vi "Set Information Panel Position.vi"(9 "Show":bool, 10 "Docs Subpanel":refnum<vi>, 11 "VI in":refnum<vi>) -> (0 "error out":errorcluster)   [LabVIEW 2019, in "Panther Dashboard.lvlib"]
uses:
  Panther Dashboard.lvlib
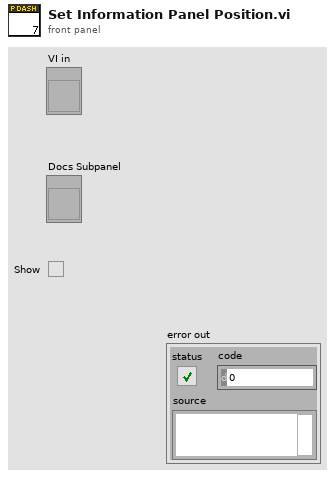
[diagram p1: front panel]
types:
  T1 = typedef "LVRectTypeDef.ctl" = cluster{"Left":i16, "Top":i16, "Right":i16, "Bottom":i16}
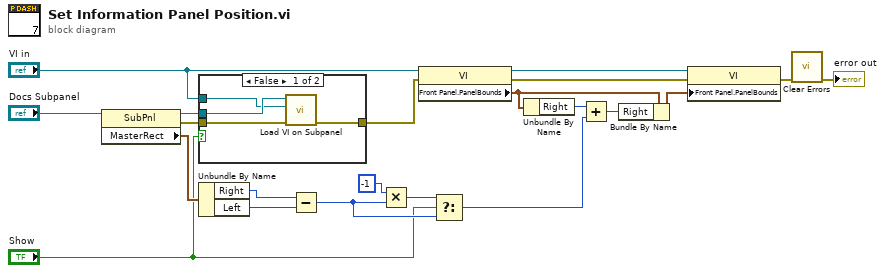
[diagram p0: block diagram]
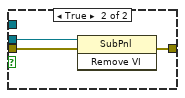
[diagram p2: hidden frame]
diagram:
  n1 = property class="SubPnl"(reference="Docs Subpanel") -> (reference out=w10:refnum<vi>, error out=w18:errorcluster, "MasterRect"=w11:T1)  [unwired: 1 in]
  n2 = case shown="False" "Show" {
    tunnel: w10 -> [w23 w26]
    tunnel: [w24 w28] -> w21
    tunnel: w18 -> [w25 w27]
    tunnel: "VI in" -> [w22 _]
    frame False {
      n3 = call "Load VI on Subpanel.vi"("error in (no error)"=w25, "VI Refnum"=w22, "Subpanel"=w23) -> ("error out"=w24:errorcluster)  [unwired: 8 in]
    }
    frame True {
      n4 = invoke class="SubPnl" method="Remove VI"(reference=w26, error in=w27) -> (error out=w28:errorcluster)  [unwired: 1 in, 2 out]
    }
  }
  n5 = Unbundle By Name(w11) -> ("Right"=w13:i16, "Left"=w12:i16)
  n6 = Subtract(x=w13, y=w12) -> (x-y=w15:i16)
  n7 = Multiply(x=i16 -1, y=w15) -> (x*y=w14:i16)
  n8 = property class="VI"(reference="VI in", error in=w21) -> (reference out=w3:refnum<vi>, error out=w19:errorcluster, "Front Panel.PanelBounds"=w4:T1)
  n9 = Select(t=w14, s="Show", f=w15) -> (s? t:f=w8:i16)
  n10 = Unbundle By Name(w4) -> ("Right"=w6:i16)
  n11 = Add(x=w6, y=w8) -> (x+y=w7:i16)
  n12 = Bundle By Name(cluster=w4, "Right"=w7) -> (w5:T1)
  n13 = property class="VI"(reference=w3, error in=w19, "Front Panel.PanelBounds"=w5) -> (error out=w17:errorcluster)  [unwired: 1 out]
  n14 = call <vilib>:"Clear Errors.vi"("error in (no error)"=w17) -> ("error out"=→"error out":errorcluster)  [unwired: 5 in, 1 out]
